vi "TL_create_tasks_list.vi"(4 "Dt (s)":dbl, 5 "error in":errorcluster, 6 "Channel #":i32, 7 "N ROIs":i32, 8 "TL array":dbl[][](array[numeric])) -> (0 "error out":errorcluster, 3 "Task list":T1[](array[typedef]))   [LabVIEW 2015]
uses:
  CONTROLS/Q_main_element.ctl
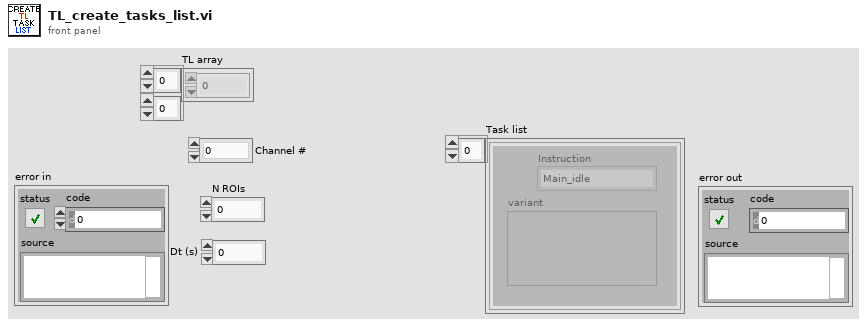
[diagram p1: front panel]
types:
  T1 = typedef "Q_main_element.ctl" = cluster{"variant":variant, "Instruction":enum16{"Main_idle", "Main_initialize", "Main_initialize_TDMS", "Main_initialize_Queue", "Main_error", "Main_DAQ_initialization_results", "Main_ASI_initialization_results", "Main_Piezo_initialization_results", "Main_Valve_initialization_results", "Main_Pump_initialization_results", "Main_CAMERA_initialization_results", "Main_DAQ_error", "Main_ASI_error", "Main_Piezo_error", "Main_CAMERA_error", "Main_Valve_error", "Main_Pump_error", "Main_start_acquiring", "Main_not_acquiring", "Main_acquiring", "Main_stop_acquiring", "Main_change_exposure", "Main_change_z_scan_parameters", "Main_define_ROI", "Main_read_kinetic_time", "Main_cooler", "Main_read_temperature", "Main_save_XY", "Main_load_XY", "Main_discard_XY", "Main_move_to_XY", "Main_measure_QPD", "Main_autofocus_calibration", "Main_save_PID", "Main_change_H_valve_position", "Main_two_way_valve", "Main_save_movie", "Main_init_single_scan", "Main_single_scan", "Main_stop_single_scan", "Main_merFISH_illumination_parameters", "Main_merFISH_buffer_probe_list", "Main_merFISH_injections_procedure", "Main_merFISH_save_setpoint", "Main_merFISH_init", "Main_merFISH_resume", "Main_merFISH_start_autofocus", "Main_merFISH_open_close_valve_merFISH", "Main_merFISH_open_close_valve_photobleaching", "Main_merFISH_hybridization", "Main_merFISH_move_to_ROI", "Main_merFISH_wait_stabilization", "Main_merFISH_scan", "Main_merFISH_photobleaching_injection", "Main_merFISH_photobleaching", "Main_merFISH_save", "Main_merFISH_send_email", "Main_merFISH_close", "Main_TL_define_parameters", "Main_TL_init", "Main_TL_start_autofocus", "Main_TL_move_to_ROI", "Main_TL_wait_for_stabilization", "Main_TL_scan", "Main_TL_wait_cycle_end", "Main_TL_close", "Main_STOP"}}
  T2 = cluster{"i":i32, "data":cluster{"Channel":string, "ROI #":i32}}
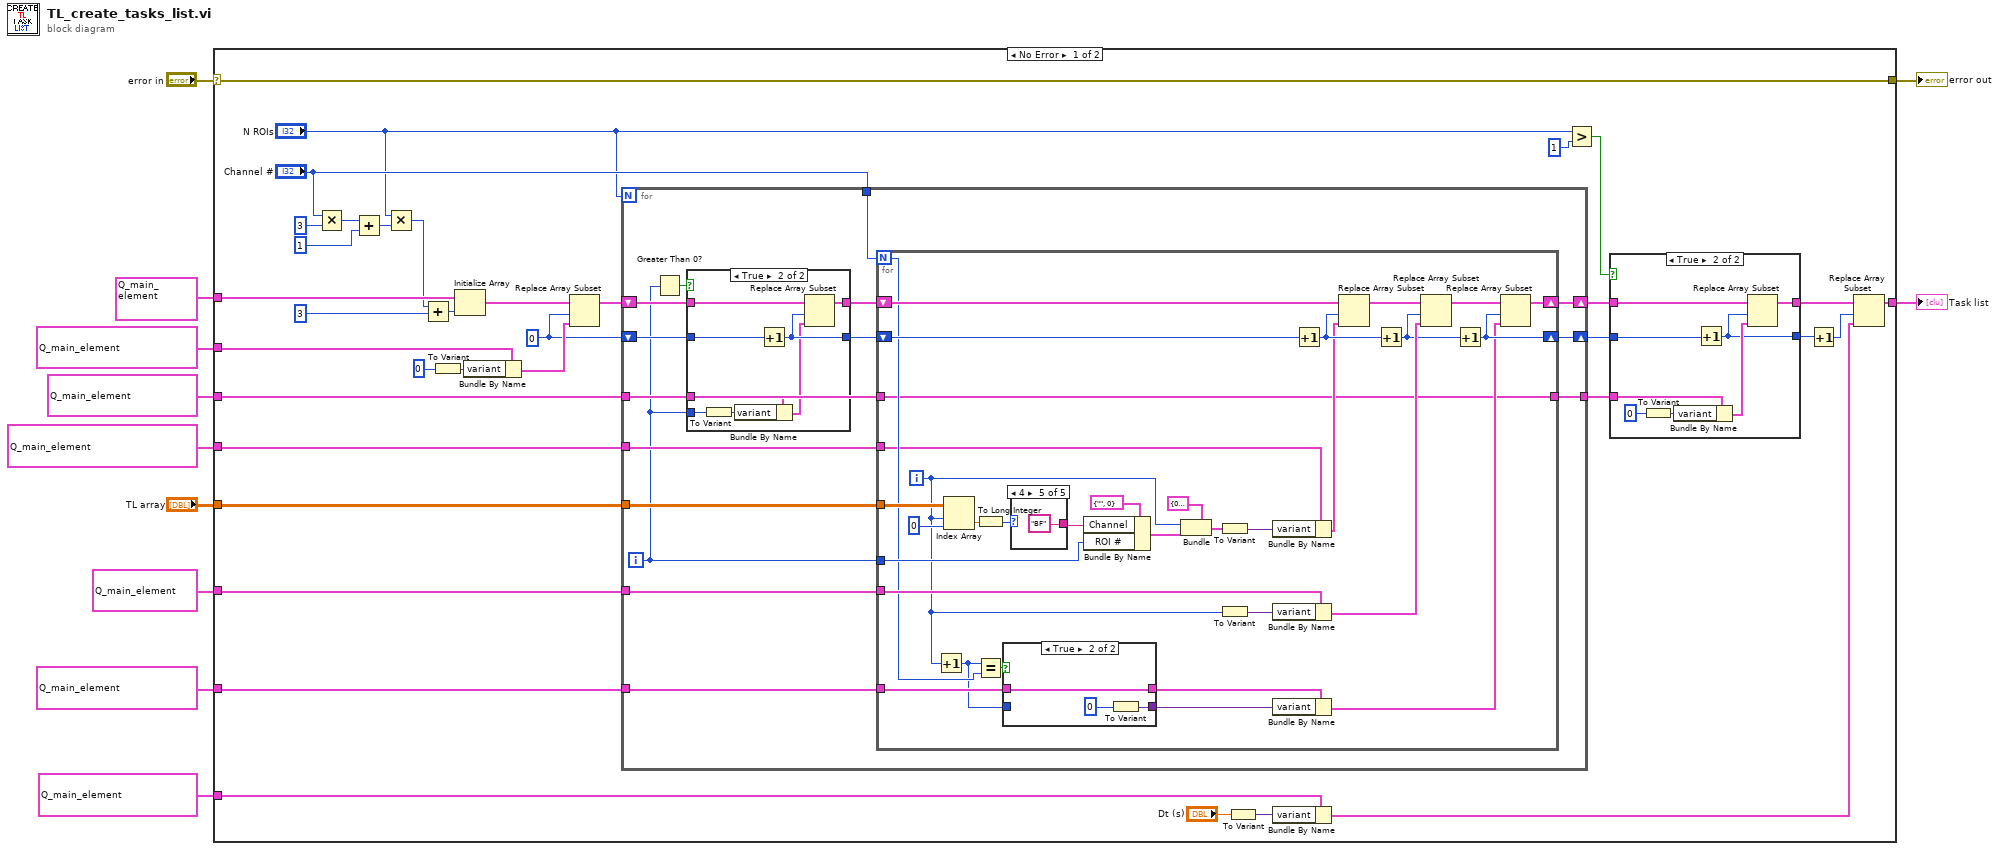
[diagram p0: block diagram]
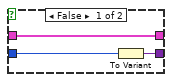
[diagram p4: hidden frame]
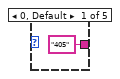
[diagram p5: hidden frame]
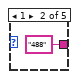
[diagram p6: hidden frame]
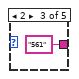
[diagram p7: hidden frame]
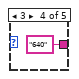
[diagram p8: hidden frame]
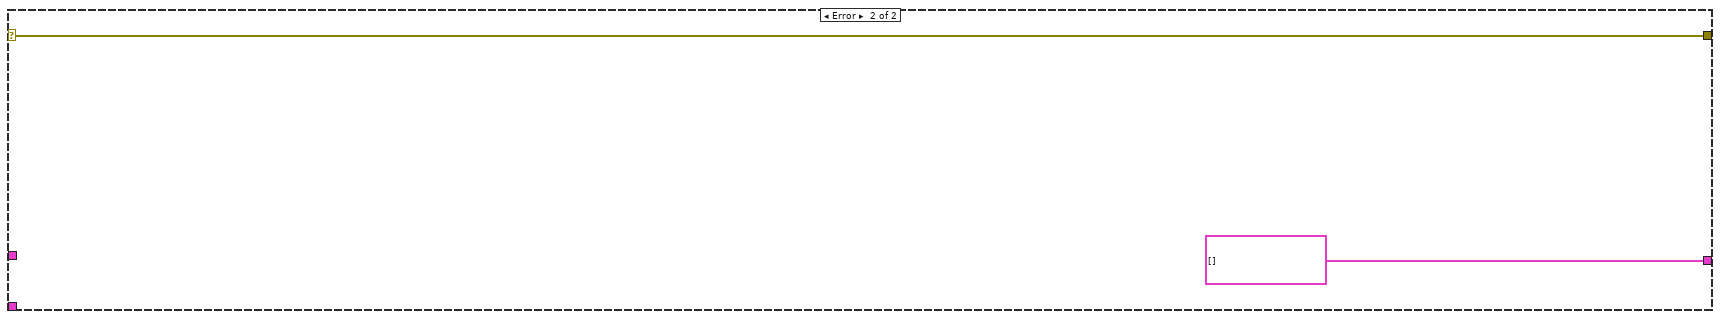
[diagram p9: hidden frame]
diagram:
  n1 = case shown="No Error" "error in" {
    selector: "error in" -> [w22 w127]
    tunnel: [w31 T1[] []] -> w11
    tunnel: T1 {"variant"=variant, "Instruction"=enum."Main_idle"} ("element") -> [w45 _]
    tunnel: T1 {"variant"=variant, "Instruction"=enum."Main_TL_wait_for_stabilization"} ("element") -> [w44 _]
    tunnel: T1 {"variant"=variant, "Instruction"=enum."Main_TL_scan"} ("element") -> [w43 _]
    tunnel: T1 {"variant"=variant, "Instruction"=enum."Main_TL_move_to_ROI"} ("element") -> [w38 _]
    tunnel: T1 {"variant"=variant, "Instruction"=enum."Main_TL_wait_cycle_end"} ("element") -> [w41 _]
    tunnel: T1 {"variant"=variant, "Instruction"=enum."Main_TL_start_autofocus"} ("element") -> [w35 _]
    tunnel: "TL array" -> [w23 _]
    tunnel: [w22 w127] -> w2
    tunnel: T1 {"variant"=variant, "Instruction"=enum."Main_TL_start_autofocus"} ("element") -> [w20 _]
    frame No Error {
      w21 = 0 ("index")
      n2 = Multiply(x="Channel #", y=3) -> (x*y=w29:i32)
      n3 = Add(x=w29, y=1) -> (x+y=w26:i32)
      n4 = Multiply(x="N ROIs", y=w26) -> (x*y=w27:i32)
      n5 = Add(x=w27, y=3) -> (x+y=w42:i32)
      n6 = To Variant(anything=0 ("index (row)")) -> (Variant=w33:variant)
      n7 = Initialize Array(w45, w42) -> (w37:T1[])
      n8 = Bundle By Name(cluster=w35, "variant"=w33) -> (w34:T1)
      n9 = Replace Array Subset(array=w37, new element=w34, index=w21) -> (w36:T1[])
      n10 = for {
        N: "N ROIs" -> [_]
        shift-right: [w69] -> w18
        shift-left: w36 -> [w64]
        tunnel: w44 -> [w67]
        tunnel: w43 -> [w66]
        shift-right: [w70] -> w16
        shift-left: w21 -> [w65]
        tunnel: w38 -> [w60]
        tunnel: "Channel #" -> [w68]
        tunnel: w23 -> [w63]
        tunnel: w20 -> [w62]
        tunnel: [w61] -> w19
        i -> [w58]
        n11 = Greater Than 0?(x=w58) -> (x > 0?=w59:bool)
        n12 = case shown="True" w59 {
          tunnel: [w74 w82] -> w72
          tunnel: [w73 w81] -> w71
          tunnel: w65 -> [w73 w80]
          tunnel: w64 -> [w74 w79]
          tunnel: w58 -> [_ w77]
          tunnel: w60 -> [_ w75]
          frame False {
          }
          frame True {
            n13 = To Variant(anything=w77) -> (Variant=w78:variant)
            n14 = Bundle By Name(cluster=w75, "variant"=w78) -> (w76:T1)
            n15 = Increment(x=w80) -> (x+1=w81:i32)
            n16 = Replace Array Subset(array=w79, new element=w76, index=w81) -> (w82:T1[])
          }
        }
        n17 = for {
          N: w68 -> [w94]
          shift-right: [w101] -> w69
          shift-left: w72 -> [w102]
          shift-right: [w100] -> w70
          shift-left: w71 -> [w103]
          tunnel: w67 -> [w90]
          tunnel: w66 -> [w105]
          tunnel: w63 -> [w113]
          tunnel: w58 -> [w108]
          tunnel: w62 -> [w98]
          tunnel: [w83] -> w61
          tunnel: w60 -> [w83]
          i -> [w87]
          n18 = Increment(x=w87) -> (x+1=w93:i32)
          n19 = Index Array(array=w113, index (row)=w87, index (col)=0 ("disabled index (col)")) -> (element=w111:dbl)
          n20 = To Long Integer(number=w111) -> (32bit integer=w110:i32)
          n21 = Equal?(x=w93, y=w94) -> (x = y?=w99:bool)
          n22 = case shown="True" w99 {
            tunnel: w98 -> [w118 w121]
            tunnel: [w118 w121] -> w97
            tunnel: [w117 w120] -> w95
            tunnel: w93 -> [w116 _]
            frame False {
              n23 = To Variant(anything=w116) -> (Variant=w117:variant)
            }
            frame True {
              n24 = To Variant(anything=0 ("disabled index (col)")) -> (Variant=w120:variant)
            }
          }
          n25 = case shown="4" w110 {
            tunnel: ["405" "488" "561" "640" "BF"] -> w109
            frame 0, Default {
            }
            frame 1 {
            }
            frame 2 {
            }
            frame 3 {
            }
            frame 4 {
            }
          }
          n26 = Bundle By Name(cluster=cluster{"Channel":string, "ROI #":i32} {"Channel"="", "ROI #"=0} ("data"), "Channel"=w109, "ROI #"=w108) -> (w86:cluster{"Channel":string, "ROI #":i32})
          n27 = Bundle(cluster=T2 {"i"=0, "data"={"Channel"="", "ROI #"=0}} ("output cluster"), "i"=w87, "data"=w86) -> (w85:T2)
          n28 = To Variant(anything=w85) -> (Variant=w107:variant)
          n29 = To Variant(anything=w87) -> (Variant=w106:variant)
          n30 = Bundle By Name(cluster=w90, "variant"=w107) -> (w89:T1)
          n31 = Bundle By Name(cluster=w105, "variant"=w106) -> (w104:T1)
          n32 = Bundle By Name(cluster=w97, "variant"=w95) -> (w96:T1)
          n33 = Increment(x=w103) -> (x+1=w114:i32)
          n34 = Replace Array Subset(array=w102, new element=w89, index=w114) -> (w115:T1[])
          n35 = Increment(x=w114) -> (x+1=w92:i32)
          n36 = Replace Array Subset(array=w115, new element=w104, index=w92) -> (w91:T1[])
          n37 = Increment(x=w92) -> (x+1=w100:i32)
          n38 = Replace Array Subset(array=w91, new element=w96, index=w100) -> (w101:T1[])
        }
      }
      n39 = To Variant(anything="Dt (s)") -> (Variant=w40:variant)
      n40 = Bundle By Name(cluster=w41, "variant"=w40) -> (w39:T1)
      n41 = Greater?(x="N ROIs", y=1) -> (0:w12:bool)
      n42 = case shown="True" w12 {
        tunnel: w19 -> [_ w56]
        tunnel: w18 -> [w49 w54]
        tunnel: [w49 w53] -> w17
        tunnel: w16 -> [w48 w52]
        tunnel: [w48 w50] -> w15
        frame False {
        }
        frame True {
          n43 = To Variant(anything=0 ("index (row)")) -> (Variant=w57:variant)
          n44 = Bundle By Name(cluster=w56, "variant"=w57) -> (w51:T1)
          n45 = Increment(x=w52) -> (x+1=w50:i32)
          n46 = Replace Array Subset(array=w54, new element=w51, index=w50) -> (w53:T1[])
        }
      }
      n47 = Increment(x=w15) -> (x+1=w46:i32)
      n48 = Replace Array Subset(array=w17, new element=w39, index=w46) -> (w31:T1[])
    }
    frame Error {
    }
  }
  "Task list" <- w11
  "error out" <- w2
